vi "FDD Self TRAINING Polynomial APPLY FIT Ver02.vi"(7 "Polynomial ORDER\n(1st, 2nd, or 3rd)":i32=1, 9 "Which Model?\n(Row # = 0 to N)":i32=32, 10 "Independent Variables \n(3 values = Tid, Tidp, Tod)":dbl[](array[numeric])=[80.0, 60.5, 95.0], 11 "Coefficients with MSE File Path":path=path "C:/Vance/FDD Split System Project/FDD_LOW-HIGH_EfficiencyHP_Testing/Airtemp 16SEER/SHORT LINESET DATA/NF Cool Short/Airtemp-NF-Cool-Short-3rdOrder-FullCoeff.txt") -> (1 "ONLY Coefficients Array - Numeric":dbl[](array[numeric]) format="%_4p", 2 "Dependent Variable NAME":string, 3 "Calculated or Predicted VALUE":dbl)   [LabVIEW 2017]
uses:
  <vilib>/Utility/file.llb/Read Delimited Spreadsheet (string).vi
panel:
  in  "Tab Control":enum32{"INPUT Filename #1"}(tab)
  out "Coefficients Array - String":string[][](array[string])=[["ID_Xitron_Amps", "3.649182597E+0", "-5.140536303E-2", "2.881361728E-2", "-1.646757582E-2", "-2.402508606E-3", "6.602898885E-4", "4.179192017E-4", "1.267049882E-3", "6.501088333E-4", "-2.620550058E-4", "6.653976606E-6", "-1.708698056E-5", "8.692189159E-7", "-3.833312073E-6", "2.400456481E-5", "-8.196342284E-6", "-1.867608948E-6", "-8.415340803E-6", "5.486740068E-6", "1.699011560E-6", "9.690230426E-5", "6.880000000E+2", "1.963418024E+0", "1.932768441E-2"], ["ID_Xitron_Watts", "1.716229164E+2", "4.524054493E+0", "5.220102345E+0", "6.418177038E+0", "4.290692245E-2", "1.821805238E-2", "-1.124104457E-2", "-8.824969946E-2", "-1.166961761E-1", "-7.952292636E-2", "-1.422440795E-3", "-3.133902282E-3", "3.751462955E-4", "-5.178701767E-4", "2.536101609E-3", "-2.843734293E-5", "1.781301284E-3", "-1.484115870E-4", "1.368702178E-3", "3.084720061E-4", "6.243538110E+0", "6.880000000E+2", "1.963418024E+0", "4.906006925E+0"], ["OD_Xitron_Amps", "-2.013666809E+1", "5.895639722E-1", "-6.152918631E-1", "7.416404081E-1", "2.429300648E-2", "-3.985684156E-3", "1.199277373E-3", "-1.499044360E-2", "-5.428978683E-3", "-6.175574441E-3", "-8.599564404E-5", "1.423009400E-4", "-3.931088897E-7", "4.392436604E-5", "-2.108058706E-4", "5.559595816E-5", "-1.953419081E-5", "9.765111857E-5", "-3.027109034E-5", "1.631585602E-5", "8.721957263E-3", "6.880000000E+2", "1.963418024E+0", "1.833663966E-1"], ["OD_Xitron_Watts", "-6.618108354E+3", "1.891326198E+2", "-1.519041438E+2", "1.957588852E+2", "7.170307753E+0", "-9.645787016E-1", "1.489837836E-1", "-4.769126088E+0", "-1.974786395E+0", "-1.581263304E+0", "-2.906099271E-2", "3.417145482E-2", "-4.089114264E-4", "9.815585226E-3", "-5.541768764E-2", "1.721648401E-2", "2.694563150E-3", "2.858072095E-2", "-6.579645117E-3", "4.327883084E-3", "4.748946922E+2", "6.880000000E+2", "1.963418024E+0", "4.278696001E+1"], ["1500_ODLiqSV_TempF", "-4.585568082E+1", "-3.179944862E-1", "6.709568073E-1", "2.558442973E+0", "-4.709548642E-2", "-8.077274201E-2", "-8.182564700E-3", "6.900856647E-2", "2.520637506E-2", "1.959412419E-2", "5.772469079E-4", "-6.760434357E-4", "3.261229720E-4", "-1.822958171E-5", "4.383995310E-4", "-9.638001637E-5", "-2.762269210E-4", "-3.447483842E-4", "3.281085348E-4", "-1.568674968E-4", "3.605191728E-1", "6.880000000E+2", "1.963418024E+0", "1.178899969E+0"], ["1510_ODVapSV_TempF", "-2.524981499E+2", "3.035027022E+1", "-2.517284187E+0", "-1.349499227E+1", "3.021069222E-1", "2.235201575E-1", "-4.653221591E-2", "-6.587678304E-1", "-1.080220631E-1", "6.763840712E-2", "-7.302086758E-4", "3.834999590E-3", "-1.454390445E-3", "5.420993761E-4", "-4.426345241E-3", "5.802409144E-4", "5.233492767E-6", "3.808583702E-3", "-1.067181551E-3", "4.966372604E-5", "1.200077250E+0", "6.880000000E+2", "1.963418024E+0", "2.150885911E+0"], ["1526_Coriolis_IDSide_TempF", "-4.842315094E+1", "-1.103822645E-2", "3.773947647E-1", "2.588770976E+0", "-2.369077200E-2", "-8.280076735E-2", "-1.301817401E-2", "5.661397296E-2", "1.915600465E-2", "2.167109261E-2", "5.012325826E-4", "-5.938059862E-4", "3.075223820E-4", "3.011275874E-5", "2.667496862E-4", "-3.102377360E-5", "-2.587105277E-4", "-2.707606112E-4", "3.144593611E-4", "-1.699168272E-4", "3.367036994E-1", "6.880000000E+2", "1.963418024E+0", "1.139296380E+0"], ["1527_Coriolis_ODSide_TempF", "-5.243166565E+1", "1.029193229E-1", "9.742497441E-2", "2.826302948E+0", "-2.017037639E-3", "-8.593134019E-2", "-1.770234558E-2", "4.826595897E-2", "1.396850518E-2", "2.185245594E-2", "4.654432525E-4", "-5.437203584E-4", "3.009641069E-4", "7.553804404E-5", "1.063096855E-4", "1.096634779E-5", "-2.646547894E-4", "-2.080889222E-4", "3.223579627E-4", "-1.785506404E-4", "3.423572826E-1", "6.880000000E+2", "1.963418024E+0", "1.148821511E+0"], ["1600_IDVap_TempF", "-4.934301357E+2", "3.264320247E+1", "-2.450456574E+0", "-7.460325466E+0", "3.193026724E-1", "1.770472275E-1", "3.782493361E-2", "-6.704131915E-1", "-1.820543392E-1", "-7.019679136E-3", "-3.902996317E-4", "4.601575241E-3", "-1.267944176E-3", "3.035333565E-4", "-5.225256056E-3", "5.364605041E-4", "-5.465768990E-4", "4.062916107E-3", "-7.696228870E-4", "3.153040768E-4", "1.813312397E+0", "6.880000000E+2", "1.963418024E+0", "2.643924740E+0"], ["1601_IDLiq_TempF", "-4.844143438E+1", "-1.353672384E+0", "6.340211288E-1", "3.444826992E+0", "-6.479678449E-2", "-9.163893289E-2", "3.542190393E-3", "9.719177283E-2", "2.786507490E-2", "1.054005407E-2", "5.668761705E-4", "-7.055927749E-4", "4.053566153E-4", "-7.801185190E-5", "5.860490894E-4", "-1.169524253E-4", "-2.738485141E-4", "-5.022961589E-4", "3.245408642E-4", "-1.336724307E-4", "3.378593597E-1", "6.880000000E+2", "1.963418024E+0", "1.141249895E+0"], ["1602_ID2phase_Cool#1_TempF", "-2.066482712E+1", "2.196493252E+1", "-7.685685179E+0", "-1.189628617E+1", "6.594946945E-1", "1.214113511E-1", "-2.660448480E-1", "-6.263892498E-1", "-6.433460146E-2", "1.636241470E-1", "-7.528805413E-4", "2.690559273E-3", "-1.312521872E-3", "1.539626735E-3", "-6.085814059E-3", "1.103740516E-3", "3.629607856E-4", "3.949749020E-3", "-1.003220488E-3", "-5.598805433E-4", "4.129112078E-1", "6.880000000E+2", "1.963418024E+0", "1.261656441E+0"], ["1603_ID2Phase_Cool#2_TempF", "-4.015458109E+1", "2.280770805E+1", "-7.004230454E+0", "-1.227787951E+1", "6.260731973E-1", "1.176270768E-1", "-2.644515591E-1", "-6.234889761E-1", "-5.667946741E-2", "1.688356434E-1", "-5.731796195E-4", "2.560563959E-3", "-1.266847643E-3", "1.501411224E-3", "-5.874986140E-3", "1.003626875E-3", "2.919997628E-4", "3.928566670E-3", "-9.474044413E-4", "-5.825450754E-4", "3.877979605E-1", "6.880000000E+2", "1.963418024E+0", "1.222687673E+0"], ["1608_CompSuct_TempF", "-1.528094930E+2", "2.268345345E+1", "-1.023051056E+0", "-1.130267312E+1", "1.830036560E-1", "1.983583254E-1", "1.875691145E-3", "-4.950546158E-1", "-9.973535247E-2", "4.205611369E-2", "-6.233643553E-4", "3.071139618E-3", "-1.230773089E-3", "3.059749580E-4", "-3.099060472E-3", "4.172570843E-4", "-1.160275146E-4", "2.806841014E-3", "-7.131103906E-4", "1.289623237E-4", "9.760337296E-1", "6.880000000E+2", "1.963418024E+0", "1.939747436E+0"], ["1612_OD2PhaseHeat_F", "1.375343259E+2", "-1.904127868E+1", "6.911947135E+0", "7.356332861E+0", "-5.790635155E-1", "-1.147352753E-1", "1.644185127E-1", "5.583315256E-1", "1.246986298E-1", "-7.434084759E-2", "4.503154807E-4", "-6.333596685E-4", "1.003436680E-3", "-1.161049007E-3", "4.021066421E-3", "-6.130447944E-4", "1.039734667E-4", "-3.293007960E-3", "-4.350316849E-4", "2.344132111E-4", "1.983231695E-1", "6.880000000E+2", "1.963418024E+0", "8.743785612E-1"], ["1617_CompDisch_TempF", "-4.619956835E+2", "-2.796811999E+1", "7.558890200E+0", "3.599432317E+1", "-1.049328395E+0", "-2.112837974E-1", "6.513567757E-1", "9.196069356E-1", "6.552854782E-3", "-4.881903969E-1", "4.912137984E-4", "-1.121596795E-3", "2.282827065E-3", "-3.108662281E-3", "7.903435127E-3", "-1.686642956E-3", "-1.077725156E-3", "-5.559272560E-3", "9.706924146E-4", "1.804316884E-3", "3.519191250E+0", "6.880000000E+2", "1.963418024E+0", "3.683275532E+0"], ["1618_ID2Phase_Heat#2_F", "-1.828882612E+2", "2.509970551E+1", "-7.940743048E+0", "-8.422210484E+0", "8.744043084E-1", "1.655278777E-1", "-3.040610727E-1", "-7.805080692E-1", "-1.729566299E-1", "1.176670095E-1", "-2.019963728E-3", "3.708678881E-3", "-1.698173571E-3", "2.016372434E-3", "-7.534515923E-3", "1.770324385E-3", "7.482073657E-4", "4.749696506E-3", "-9.968740596E-4", "-3.827950439E-4", "9.121747188E-1", "6.880000000E+2", "1.963418024E+0", "1.875218113E+0"], ["1622_OD2PhaseCool_F", "-1.079342555E+2", "-5.681728059E+0", "-8.985853634E-1", "9.749367935E+0", "-1.187239790E-1", "-1.464367724E-2", "9.136074437E-2", "1.369001626E-1", "2.040683598E-2", "-1.168600191E-1", "9.787150928E-5", "4.920940653E-4", "6.320240761E-4", "-5.214726841E-4", "4.192037397E-4", "-6.977200405E-4", "-3.144420451E-5", "-4.815767216E-4", "-3.340869975E-4", "3.517868544E-4", "2.801887516E-1", "6.880000000E+2", "1.963418024E+0", "1.039293286E+0"], ["1630_ID2Phase_Heat#1_F", "1.036958015E+2", "1.854107232E+1", "-8.020385580E+0", "-1.292851450E+1", "5.907548840E-1", "1.423593049E-1", "-2.567838332E-1", "-5.666990955E-1", "-2.406262724E-2", "1.634546527E-1", "-1.028621256E-3", "2.194891794E-3", "-1.286210456E-3", "1.496264653E-3", "-5.163064752E-3", "1.045815743E-3", "5.088718207E-4", "3.491311260E-3", "-1.028752295E-3", "-5.551862467E-4", "4.653410073E-1", "6.880000000E+2", "1.963418024E+0", "1.339363428E+0"], ["1701_ODVapSV_psia", "-1.271507113E+2", "5.310358071E+1", "-1.955768746E+1", "-2.400134640E+1", "1.594268954E+0", "2.275501101E-1", "-5.951900834E-1", "-1.479095419E+0", "-1.843089529E-1", "3.564233424E-1", "-2.119399498E-3", "7.488742584E-3", "-2.760788831E-3", "3.551477869E-3", "-1.520052902E-2", "2.723027549E-3", "9.394153082E-4", "9.487891380E-3", "-2.727524957E-3", "-1.291668941E-3", "2.843216624E+0", "6.880000000E+2", "1.963418024E+0", "3.310684140E+0"], ["1702_ODLiqSV_psia", "-5.422342138E+2", "-1.159762766E+1", "-9.682897958E+0", "3.621663251E+1", "-2.044450193E-1", "-1.698402086E-1", "3.878130436E-1", "3.478059303E-1", "-5.770577163E-3", "-4.063691684E-1", "-7.496911760E-4", "9.895719005E-4", "1.421382637E-3", "-1.123470635E-3", "1.301987273E-3", "-4.470680195E-4", "-9.642171894E-4", "-1.771527599E-3", "-6.900656164E-5", "1.386338471E-3", "5.762628526E+0", "6.880000000E+2", "1.963418024E+0", "4.713278321E+0"], ["1707_IDVap_psia", "1.615316803E+1", "4.780594061E+1", "-1.545593179E+1", "-2.692720176E+1", "1.318538879E+0", "2.430331131E-1", "-5.470768080E-1", "-1.307845509E+0", "-1.197262601E-1", "3.648317280E-1", "-1.273587466E-3", "6.035640496E-3", "-2.661453376E-3", "3.112833691E-3", "-1.279419243E-2", "2.173173019E-3", "6.597065544E-4", "8.332254530E-3", "-2.269940886E-3", "-1.249089829E-3", "1.831320683E+0", "6.880000000E+2", "1.963418024E+0", "2.657020919E+0"], ["1710_ODSuctPort_psia", "5.025635613E+1", "5.002192336E+1", "-1.645924711E+1", "-2.924561169E+1", "1.405938578E+0", "2.767761540E-1", "-5.854707943E-1", "-1.392954167E+0", "-1.271941973E-1", "3.881228857E-1", "-1.348200830E-3", "6.082163940E-3", "-2.893492574E-3", "3.335508771E-3", "-1.337802658E-2", "2.262468565E-3", "6.860373423E-4", "8.828223314E-3", "-2.267542460E-3", "-1.314338024E-3", "2.069758435E+0", "6.880000000E+2", "1.963418024E+0", "2.824701783E+0"], ["1712_RotoMass_Massflow_lb/min", "-4.947722970E+1", "-3.775514116E+0", "-6.243587911E-1", "5.099321237E+0", "-6.647103644E-2", "-5.736972490E-2", "3.936854184E-2", "1.120381362E-1", "2.386415610E-2", "-4.352415740E-2", "2.096786191E-4", "1.114833845E-5", "3.710057398E-4", "-1.951028542E-4", "3.259716238E-4", "-1.557101471E-4", "-1.629776950E-4", "-5.233893635E-4", "-6.784336866E-5", "9.419508429E-5", "3.694656438E-2", "6.880000000E+2", "1.963418024E+0", "3.773981817E-1"], ["1713_RotoMass_Density_lbm/ft3", "6.972746898E+1", "5.329404135E-3", "-1.020933614E-3", "1.456172676E-3", "6.235853826E-5", "2.817350025E-5", "-7.354205153E-6", "-1.190081875E-4", "-1.498390594E-5", "-2.506210771E-5", "-3.415818956E-7", "8.689883626E-7", "-2.032567531E-7", "1.813567032E-7", "-8.362482712E-7", "1.932899152E-7", "6.608777585E-9", "6.614476248E-7", "-3.338571025E-7", "1.050118285E-7", "1.959109698E-7", "6.880000000E+2", "1.963418024E+0", "8.690447708E-4"], ["1724_IDLiq_psia", "-7.379310853E+2", "-2.817639301E+0", "-1.536492625E+1", "3.897973985E+1", "2.439076392E-1", "-1.509061218E-1", "2.953041679E-1", "4.267550291E-2", "-1.174240967E-1", "-4.142987132E-1", "-2.225403189E-3", "3.035192380E-3", "1.014478034E-3", "-3.088712310E-4", "-2.342670918E-3", "4.917734818E-4", "-4.737072015E-4", "1.402022438E-4", "-6.372076570E-4", "1.348374932E-3", "9.064058769E+0", "6.880000000E+2", "1.963418024E+0", "5.911179260E+0"], ["2219_NozTemp#1_F", "-1.754312882E+1", "1.374900200E+1", "-3.317343563E+0", "-7.770249170E+0", "3.179852436E-1", "1.037596492E-1", "-1.353724228E-1", "-3.643811409E-1", "-3.212616106E-2", "8.317630275E-2", "-5.199186267E-4", "1.729729139E-3", "-8.856288738E-4", "7.884642558E-4", "-3.186354143E-3", "6.139404982E-4", "2.404447950E-4", "2.194895571E-3", "-6.576816644E-4", "-2.204444687E-4", "1.566409833E-1", "6.880000000E+2", "1.963418024E+0", "7.770795388E-1"], ["2220_NozTemp#2_F", "-1.813162554E+1", "1.372464929E+1", "-3.329206860E+0", "-7.720651535E+0", "3.153119443E-1", "1.028214455E-1", "-1.340494561E-1", "-3.624910582E-1", "-3.119921692E-2", "8.260349684E-2", "-4.950354594E-4", "1.695214482E-3", "-8.807374944E-4", "7.835194513E-4", "-3.156630090E-3", "6.045147830E-4", "2.213202608E-4", "2.182689009E-3", "-6.389018610E-4", "-2.187143326E-4", "1.534357740E-1", "6.880000000E+2", "1.963418024E+0", "7.690880929E-1"], ["Exit TC Grid AVG Temp (F)", "2.499177681E+1", "1.313499641E+1", "-1.579284719E+0", "-9.751778296E+0", "2.359287146E-1", "1.185207521E-1", "-1.133913691E-1", "-3.336428953E-1", "-2.706899567E-2", "9.142140009E-2", "-6.137909095E-4", "1.874317129E-3", "-8.759602864E-4", "6.200158032E-4", "-2.701478540E-3", "5.373648669E-4", "3.741687163E-4", "1.966048660E-3", "-8.066352292E-4", "-2.146806852E-4", "1.296028769E-1", "6.880000000E+2", "1.963418024E+0", "7.068383339E-1"], ["TC Grid  DT Temp (F)", "-4.257854183E+1", "-9.590738646E+0", "1.478875346E+0", "8.352663558E+0", "-3.728266342E-1", "-1.110798530E-1", "2.543815249E-1", "3.488619787E-1", "1.191094500E-3", "-1.219780037E-1", "9.010565418E-5", "-1.961396831E-3", "1.173883695E-3", "-1.402270925E-3", "3.985703674E-3", "-7.725970486E-4", "-1.974511799E-6", "-2.262454546E-3", "8.308079870E-4", "4.062025873E-4", "4.479560438E-1", "6.880000000E+2", "1.963418024E+0", "1.314106228E+0"], ["AVG Nozzle Temp (F)", "-1.783734967E+1", "1.373682483E+1", "-3.323275076E+0", "-7.745450706E+0", "3.166485628E-1", "1.032905394E-1", "-1.347109186E-1", "-3.634360716E-1", "-3.166268813E-2", "8.288990059E-2", "-5.074770197E-4", "1.712471779E-3", "-8.831831306E-4", "7.859917415E-4", "-3.171491893E-3", "6.092276189E-4", "2.308825109E-4", "2.188792115E-3", "-6.482917459E-4", "-2.195793956E-4", "1.549526808E-1", "6.880000000E+2", "1.963418024E+0", "7.728804477E-1"], ["AVG Noz DP (in H2O)", "-1.137797681E+0", "1.139881567E-1", "-4.855784009E-2", "1.778732377E-2", "2.341579537E-3", "-5.339749034E-5", "-1.255346805E-4", "-2.466438349E-3", "-5.517348287E-4", "-1.204757019E-4", "-8.404469252E-6", "-1.104968660E-6", "-4.258171433E-7", "1.715886404E-6", "-1.068197014E-5", "3.957447596E-6", "4.043993108E-6", "1.263395541E-5", "1.739848601E-6", "1.336642894E-7", "4.743755967E-5", "6.880000000E+2", "1.963418024E+0", "1.352302787E-2"], ["Unit ESP (in H2O)", "-3.439738970E+0", "2.916621869E-1", "-1.240495672E-1", "-3.041133172E-2", "5.885990550E-3", "-4.074613399E-4", "-5.756427155E-4", "-6.075054737E-3", "-1.119043745E-3", "7.007862690E-4", "-1.667015324E-5", "1.651625482E-8", "-1.637373039E-6", "3.626950987E-6", "-3.123506980E-5", "1.104404076E-5", "1.016745289E-5", "3.178763763E-5", "1.637571913E-6", "-2.961992416E-6", "2.398511109E-4", "6.880000000E+2", "1.963418024E+0", "3.040770481E-2"], ["Indoor Unit SCFM", "-7.335853432E+0", "3.749046443E+1", "-2.818193672E+0", "1.931921094E+1", "-2.294186759E-1", "-1.787247292E-1", "2.855866698E-1", "-3.375291253E-1", "-4.240954599E-2", "-2.309628818E-1", "-6.426877515E-4", "-7.668786554E-3", "1.823057108E-3", "-1.104643875E-3", "7.229583417E-3", "-9.636155661E-4", "-5.625477236E-5", "3.089714452E-4", "3.740617520E-3", "5.791876535E-4", "1.744373054E+1", "6.880000000E+2", "1.963418024E+0", "8.200351306E+0"], ["Indoor Unit CFM", "5.870901161E+1", "8.838692813E+1", "-5.113773977E+1", "9.405102985E-1", "2.801213135E+0", "1.122477420E-1", "-3.965379432E-1", "-2.376335379E+0", "-5.733522956E-1", "8.559257420E-2", "-8.812479176E-3", "6.164455892E-3", "-2.165085942E-3", "2.852821761E-3", "-1.864415606E-2", "5.286769922E-3", "4.632039322E-3", "1.352960052E-2", "-1.706240441E-3", "-3.905071358E-4", "3.145326437E+1", "6.880000000E+2", "1.963418024E+0", "1.101147852E+1"], ["Sensible Capacity (Btu/h)", "-9.575239359E+4", "-1.294536948E+4", "1.905086089E+3", "1.265908979E+4", "-5.378583272E+2", "-1.635344460E+2", "3.697621314E+2", "4.932746269E+2", "3.061895457E+0", "-1.822635301E+2", "2.058180973E-1", "-2.958783615E+0", "1.720283557E+0", "-2.023987174E+0", "5.796953442E+0", "-1.158494644E+0", "-6.877770687E-2", "-3.213286283E+0", "1.286961793E+0", "6.019894048E-1", "8.591656358E+5", "6.880000000E+2", "1.963418024E+0", "1.819915494E+3"], ["Latent Capacity (Btu/h)", "-1.613809630E+5", "-9.924934542E+1", "-7.112672363E+2", "5.672008031E+3", "-2.210236246E+2", "-2.203800999E+1", "5.895196575E+1", "9.658382518E+1", "1.223361300E+2", "-6.982281156E+1", "1.924945356E+0", "5.985960021E-1", "1.967482386E-1", "-2.646350109E-1", "-1.249715862E-1", "-8.319681059E-1", "-1.359122700E+0", "-9.301681808E-2", "-2.254308371E-1", "2.472010209E-1", "8.962121847E+5", "6.880000000E+2", "1.963418024E+0", "1.858738076E+3"], ["TOTAL Capacity (Btu/h)", "-2.571333565E+5", "-1.304461883E+4", "1.193818849E+3", "1.833109782E+4", "-7.588819518E+2", "-1.855724560E+2", "4.287140971E+2", "5.898584521E+2", "1.253980255E+2", "-2.520863417E+2", "2.130763453E+0", "-2.360187615E+0", "1.917031796E+0", "-2.288622185E+0", "5.671981856E+0", "-1.990462750E+0", "-1.427900407E+0", "-3.306303101E+0", "1.061530957E+0", "8.491904258E-1", "9.226341900E+5", "6.880000000E+2", "1.963418024E+0", "1.885938583E+3"], ["SHR", "1.409496581E+0", "-5.315813104E-1", "5.305446081E-2", "3.732189749E-1", "-9.538459857E-3", "-5.387729077E-3", "7.413719359E-3", "1.444159300E-2", "-1.323440633E-3", "-4.104652237E-3", "-2.791338927E-5", "-7.706918986E-5", "4.468436884E-5", "-4.215603811E-5", "1.396978807E-4", "-8.270449144E-6", "2.022935805E-5", "-9.699612686E-5", "3.204577950E-5", "1.139932919E-5", "7.667089070E-4", "6.880000000E+2", "1.963418024E+0", "5.436608099E-2"], ["ODVapSV_Suph_F", "-1.531685671E+2", "7.736125102E+0", "5.496257324E+0", "-3.831114058E+0", "-3.658565402E-1", "1.253264058E-1", "2.042712961E-1", "-3.416551092E-2", "-3.120034254E-2", "-7.719138247E-2", "1.433280389E-4", "8.685130214E-4", "-2.772884354E-4", "-9.705029207E-4", "1.836149520E-3", "-5.563934051E-4", "-3.484705855E-4", "-1.600846766E-4", "-1.082111631E-5", "5.747559901E-4", "1.466487551E+0", "6.880000000E+2", "1.963418024E+0", "2.377672111E+0"], ["ODVapSV_Tsat_F", "-9.932961364E+1", "2.261414618E+1", "-8.013541192E+0", "-9.663878230E+0", "6.679634583E-1", "9.819376864E-2", "-2.508035217E-1", "-6.246023430E-1", "-7.682171584E-2", "1.448297857E-1", "-8.735367507E-4", "2.966486689E-3", "-1.177102087E-3", "1.512602327E-3", "-6.262494796E-3", "1.136634316E-3", "3.537041316E-4", "3.968668494E-3", "-1.056360543E-3", "-5.250922350E-4", "4.597261742E-1", "6.880000000E+2", "1.963418024E+0", "1.331258485E+0"], ["ODLiqSV_Tsat_F", "-1.695480861E+2", "-3.791180368E+0", "-1.577375499E+0", "1.079483774E+1", "-8.295583575E-2", "-5.296622944E-2", "1.005231365E-1", "1.171244146E-1", "7.032719084E-4", "-1.132741136E-1", "-8.780386147E-5", "1.453020048E-4", "4.455193121E-4", "-3.667343510E-4", "5.597909886E-4", "-1.845359755E-4", "-2.104028951E-4", "-6.082820082E-4", "6.144653732E-6", "3.573211894E-4", "2.656341209E-1", "6.880000000E+2", "1.963418024E+0", "1.011939861E+0"], ["ODLiqSV_Tsub_F", "-1.236923822E+2", "-3.473185910E+0", "-2.248331979E+0", "8.236393766E+0", "-3.586032918E-2", "2.780652564E-2", "1.087056897E-1", "4.811583354E-2", "-2.450311258E-2", "-1.328682286E-1", "-6.650509763E-4", "8.213457362E-4", "1.193962742E-4", "-3.485047271E-4", "1.213912052E-4", "-8.815588413E-5", "6.582418640E-5", "-2.635335246E-4", "-3.219640274E-4", "5.141886621E-4", "1.009382009E+0", "6.880000000E+2", "1.963418024E+0", "1.972606924E+0"], ["1612_OD2phase_Heating_F", "1.375343259E+2", "-1.904127868E+1", "6.911947135E+0", "7.356332861E+0", "-5.790635155E-1", "-1.147352753E-1", "1.644185127E-1", "5.583315256E-1", "1.246986298E-1", "-7.434084759E-2", "4.503154807E-4", "-6.333596685E-4", "1.003436680E-3", "-1.161049007E-3", "4.021066421E-3", "-6.130447944E-4", "1.039734667E-4", "-3.293007960E-3", "-4.350316849E-4", "2.344132111E-4", "1.983231695E-1", "6.880000000E+2", "1.963418024E+0", "8.743785612E-1"], ["1622_OD2phase_Cooling_F", "-1.079342555E+2", "-5.681728059E+0", "-8.985853634E-1", "9.749367935E+0", "-1.187239790E-1", "-1.464367724E-2", "9.136074437E-2", "1.369001626E-1", "2.040683598E-2", "-1.168600191E-1", "9.787150928E-5", "4.920940653E-4", "6.320240761E-4", "-5.214726841E-4", "4.192037397E-4", "-6.977200405E-4", "-3.144420451E-5", "-4.815767216E-4", "-3.340869975E-4", "3.517868544E-4", "2.801887516E-1", "6.880000000E+2", "1.963418024E+0", "1.039293286E+0"], ["1710_CompSuct_psia", "5.025635613E+1", "5.002192336E+1", "-1.645924711E+1", "-2.924561169E+1", "1.405938578E+0", "2.767761540E-1", "-5.854707943E-1", "-1.392954167E+0", "-1.271941973E-1", "3.881228857E-1", "-1.348200830E-3", "6.082163940E-3", "-2.893492574E-3", "3.335508771E-3", "-1.337802658E-2", "2.262468565E-3", "6.860373423E-4", "8.828223314E-3", "-2.267542460E-3", "-1.314338024E-3", "2.069758435E+0", "6.880000000E+2", "1.963418024E+0", "2.824701783E+0"], ["CompSuct_TempF", "-1.528094930E+2", "2.268345345E+1", "-1.023051056E+0", "-1.130267312E+1", "1.830036560E-1", "1.983583254E-1", "1.875691145E-3", "-4.950546158E-1", "-9.973535247E-2", "4.205611369E-2", "-6.233643553E-4", "3.071139618E-3", "-1.230773089E-3", "3.059749580E-4", "-3.099060472E-3", "4.172570843E-4", "-1.160275146E-4", "2.806841014E-3", "-7.131103906E-4", "1.289623237E-4", "9.760337296E-1", "6.880000000E+2", "1.963418024E+0", "1.939747436E+0"], ["CompSuct_Suph_F", "-1.340849531E+2", "1.552772665E+0", "5.795097431E+0", "5.883809093E-1", "-4.037199694E-1", "8.091812283E-2", "2.472291050E-1", "8.887894393E-2", "-4.934879950E-2", "-1.166015906E-1", "-5.477045901E-5", "6.352853249E-4", "-1.064105490E-5", "-1.102997392E-3", "2.418734469E-3", "-5.272020758E-4", "-3.825618854E-4", "-8.687979975E-4", "1.998307055E-4", "6.662056741E-4", "1.229631082E+0", "6.880000000E+2", "1.963418024E+0", "2.177209345E+0"], ["CompSuct_Tsat_F", "-1.872454573E+1", "2.113068173E+1", "-6.818149392E+0", "-1.189105404E+1", "5.867236285E-1", "1.174402184E-1", "-2.453534060E-1", "-5.839335832E-1", "-5.038654486E-2", "1.586576953E-1", "-5.685937675E-4", "2.435853951E-3", "-1.220132075E-3", "1.408972300E-3", "-5.517794786E-3", "9.444590541E-4", "2.665342960E-4", "3.675639121E-3", "-9.129409524E-4", "-5.372432956E-4", "3.467028339E-1", "6.880000000E+2", "1.963418024E+0", "1.156089533E+0"], ["CompDisch_psia", "-5.422342138E+2", "-1.159762766E+1", "-9.682897958E+0", "3.621663251E+1", "-2.044450193E-1", "-1.698402086E-1", "3.878130436E-1", "3.478059303E-1", "-5.770577163E-3", "-4.063691684E-1", "-7.496911760E-4", "9.895719005E-4", "1.421382637E-3", "-1.123470635E-3", "1.301987273E-3", "-4.470680195E-4", "-9.642171894E-4", "-1.771527599E-3", "-6.900656164E-5", "1.386338471E-3", "5.762628526E+0", "6.880000000E+2", "1.963418024E+0", "4.713278321E+0"], ["1617_CompDisch_TempF", "-4.619956835E+2", "-2.796811999E+1", "7.558890200E+0", "3.599432317E+1", "-1.049328395E+0", "-2.112837974E-1", "6.513567757E-1", "9.196069356E-1", "6.552854782E-3", "-4.881903969E-1", "4.912137984E-4", "-1.121596795E-3", "2.282827065E-3", "-3.108662281E-3", "7.903435127E-3", "-1.686642956E-3", "-1.077725156E-3", "-5.559272560E-3", "9.706924146E-4", "1.804316884E-3", "3.519191250E+0", "6.880000000E+2", "1.963418024E+0", "3.683275532E+0"], ["CompDisch_Suph_F", "-2.925827467E+2", "-2.417600442E+1", "9.133805026E+0", "2.519885952E+1", "-9.662875471E-1", "-1.582919624E-1", "5.508231642E-1", "8.024239119E-1", "5.848799247E-3", "-3.749389603E-1", "5.786602502E-4", "-1.266756848E-3", "1.837049851E-3", "-2.741621942E-3", "7.343150387E-3", "-1.501847674E-3", "-8.674450003E-4", "-4.950702581E-3", "9.645379653E-4", "1.447192086E-3", "2.463784998E+0", "6.880000000E+2", "1.963418024E+0", "3.081869016E+0"], ["CompDisch_Tsat_F", "-1.694129093E+2", "-3.792115026E+0", "-1.574914602E+0", "1.079546212E+1", "-8.304084171E-2", "-5.299181839E-2", "1.005336086E-1", "1.171830038E-1", "7.040499837E-4", "-1.132514255E-1", "-8.744658514E-5", "1.451600711E-4", "4.457771428E-4", "-3.670403291E-4", "5.602847449E-4", "-1.847952550E-4", "-2.102800637E-4", "-6.085698979E-4", "6.154437114E-6", "3.571247740E-4", "2.654244699E-1", "6.880000000E+2", "1.963418024E+0", "1.011540446E+0"], ["Refrig-Side Capacity_Btu/h", "-2.545361196E+5", "-1.933874326E+4", "-1.691551366E+3", "2.526788105E+4", "-3.929117778E+2", "-2.507092264E+2", "2.360320145E+2", "5.711951068E+2", "1.008249715E+2", "-2.430265178E+2", "8.147131932E-1", "2.069505690E-1", "1.791752730E+0", "-1.193649099E+0", "2.071187972E+0", "-8.658581461E-1", "-6.764703276E-1", "-2.760995386E+0", "-3.598132097E-1", "6.256628833E-1", "7.734237509E+5", "6.880000000E+2", "1.963418024E+0", "1.726718435E+3"], ["IDLiq@TXV_Tsat_F", "-2.195384759E+2", "-1.444944555E+0", "-2.807925177E+0", "1.129148253E+1", "2.490310461E-2", "-4.382800050E-2", "7.493409718E-2", "3.755061073E-2", "-2.616821150E-2", "-1.141182362E-1", "-4.071177131E-4", "6.492798586E-4", "3.238373038E-4", "-1.696134622E-4", "-3.433590188E-4", "2.749820935E-5", "-8.915693852E-5", "-1.089492776E-4", "-1.376855970E-4", "3.503565652E-4", "4.039700959E-1", "6.880000000E+2", "1.963418024E+0", "1.247921831E+0"], ["IDLiq@TXV_Tsub_F", "-1.710970854E+2", "-9.126850595E-2", "-3.441946765E+0", "7.846654376E+0", "8.969996120E-2", "4.781094846E-2", "7.139188230E-2", "-5.964125108E-2", "-5.403330499E-2", "-1.246582762E-1", "-9.739941629E-4", "1.354872800E-3", "-8.151946507E-5", "-9.160147507E-5", "-9.294085678E-4", "1.444508213E-4", "1.846917602E-4", "3.933473347E-4", "-4.622265177E-4", "4.840289567E-4", "1.230292577E+0", "6.880000000E+2", "1.963418024E+0", "2.177794894E+0"], ["IDVap_Suph_F", "-4.609486691E+2", "1.255642026E+1", "3.859272995E+0", "3.423801646E+0", "-2.243953864E-1", "7.409475948E-2", "2.646670209E-1", "-1.264606199E-1", "-1.354543238E-1", "-1.548129318E-1", "1.429221052E-4", "2.219176471E-3", "-1.527350979E-4", "-9.999740044E-4", "-1.830561674E-5", "-3.622936998E-4", "-7.982249998E-4", "6.288128842E-4", "1.322823748E-4", "8.205674934E-4", "2.120976931E+0", "6.880000000E+2", "1.963418024E+0", "2.859438405E+0"], ["IDVap_Tsat_F", "-3.248146899E+1", "2.008678244E+1", "-6.309729546E+0", "-1.088412723E+1", "5.436980787E-1", "1.029524844E-1", "-2.268420965E-1", "-5.439525928E-1", "-4.660002157E-2", "1.477932505E-1", "-5.332219795E-4", "2.382398929E-3", "-1.115209126E-3", "1.303507403E-3", "-5.206950557E-3", "8.987542433E-4", "2.516482706E-4", "3.434103337E-3", "-9.019053792E-4", "-5.052634053E-4", "3.005119595E-1", "6.880000000E+2", "1.963418024E+0", "1.076325560E+0"], ["CoriolisLiq_ID#1_Tsub_F", "-1.711153724E+2", "-1.433903936E+0", "-3.185320571E+0", "8.702711659E+0", "4.859392971E-2", "3.897277726E-2", "8.795223899E-2", "-1.906342389E-2", "-4.532421278E-2", "-1.357893238E-1", "-9.083501853E-4", "1.243085910E-3", "1.631478801E-5", "-1.997260487E-4", "-6.101091650E-4", "5.852203811E-5", "1.695535219E-4", "1.618117116E-4", "-4.521449833E-4", "5.202733727E-4", "1.232563118E+0", "6.880000000E+2", "1.963418024E+0", "2.179803560E+0"], ["CoriolisLiq_OD#2_Tsub_F", "-1.171164164E+2", "-3.894099723E+0", "-1.674800085E+0", "7.968534457E+0", "-8.093881395E-2", "3.296511348E-2", "1.182254796E-1", "6.885846056E-2", "-1.326522782E-2", "-1.351265665E-1", "-5.532469856E-4", "6.890223262E-4", "1.445551716E-4", "-4.422723967E-4", "4.534813670E-4", "-1.955023475E-4", "5.425183569E-5", "-4.001931168E-4", "-3.162132978E-4", "5.358718284E-4", "9.463956945E-1", "6.880000000E+2", "1.963418024E+0", "1.910069419E+0"], ["Blower_Heat_Btu/h", "5.855773907E+2", "1.543607393E+1", "1.781098920E+1", "2.189882005E+1", "1.463984194E-1", "6.215999473E-2", "-3.835444409E-2", "-3.011079746E-1", "-3.981673529E-1", "-2.713322247E-1", "-4.853367992E-3", "-1.069287459E-2", "1.279999160E-3", "-1.766973043E-3", "8.653178690E-3", "-9.702821406E-5", "6.077799981E-3", "-5.063803347E-4", "4.670011832E-3", "1.052506485E-3", "7.268567233E+1", "6.880000000E+2", "1.963418024E+0", "1.673929563E+1"], ["Adj_RefSide_Q_Btu/h", "-2.551216971E+5", "-1.935417935E+4", "-1.709362350E+3", "2.524598224E+4", "-3.930581761E+2", "-2.507713865E+2", "2.360703688E+2", "5.714962149E+2", "1.012231389E+2", "-2.427551855E+2", "8.195665604E-1", "2.176434451E-1", "1.790472732E+0", "-1.191882126E+0", "2.062534792E+0", "-8.657611172E-1", "-6.825481264E-1", "-2.760489007E+0", "-3.644832228E-1", "6.246103765E-1", "7.799978000E+5", "6.880000000E+2", "1.963418024E+0", "1.734041401E+3"], ["COP", "-2.237422820E+1", "-2.006160170E+0", "3.845570213E-1", "2.177207477E+0", "-9.755528939E-2", "-2.330712453E-2", "4.889353046E-2", "7.989071092E-2", "1.712595992E-2", "-2.933830713E-2", "2.698786334E-4", "-3.328218649E-4", "2.316797558E-4", "-2.695505600E-4", "7.495906407E-4", "-2.393156071E-4", "-1.701958633E-4", "-4.539659092E-4", "1.388851460E-4", "9.853982773E-5", "9.810289504E-3", "6.880000000E+2", "1.963418024E+0", "1.944704796E-1"], ["SCFM/TON", "2.455025009E+4", "3.115259398E+3", "-5.014085972E+2", "-2.940604234E+3", "8.074506047E+1", "3.111805892E+1", "-3.960570057E+1", "-9.290190901E+1", "-1.108955267E+1", "3.122193608E+1", "-1.250870592E-1", "2.355015576E-1", "-2.515316290E-1", "2.173017506E-1", "-6.506671942E-1", "1.524076341E-1", "7.720638828E-2", "5.233469183E-1", "-8.089481961E-2", "-8.860805990E-2", "1.023790810E+4", "6.880000000E+2", "1.963418024E+0", "1.986636392E+2"], ["ODAir_Exit_TempF", "-5.045051727E+1", "-1.021755477E+1", "1.853451132E+0", "9.784387973E+0", "-3.037557867E-1", "-1.063198454E-1", "1.378800428E-1", "3.236224866E-1", "5.352116366E-2", "-9.373435201E-2", "4.688536253E-4", "-6.657783717E-4", "8.350349652E-4", "-8.283972436E-4", "2.255287598E-3", "-5.038059967E-4", "-1.891893231E-4", "-1.827006539E-3", "1.055377137E-4", "2.812255200E-4", "1.247708707E-1", "6.880000000E+2", "1.963418024E+0", "6.935365860E-1"], ["ODAir_DT(F)", "-5.045051727E+1", "-1.021755477E+1", "1.853451132E+0", "8.784387973E+0", "-3.037557867E-1", "-1.063198454E-1", "1.378800428E-1", "3.236224866E-1", "5.352116366E-2", "-9.373435201E-2", "4.688536253E-4", "-6.657783717E-4", "8.350349652E-4", "-8.283972436E-4", "2.255287598E-3", "-5.038059967E-4", "-1.891893231E-4", "-1.827006539E-3", "1.055377137E-4", "2.812255200E-4", "1.247708707E-1", "6.880000000E+2", "1.963418024E+0", "6.935365860E-1"], ["LiqLine_DP(psid)", "1.956968715E+2", "-8.779988360E+0", "5.682028296E+0", "-2.763107338E+0", "-4.483526585E-1", "-1.893408673E-2", "9.250887569E-2", "3.051304274E-1", "1.116535196E-1", "7.929544805E-3", "1.475712013E-3", "-2.045620479E-3", "4.069046031E-4", "-8.145994043E-4", "3.644658191E-3", "-9.388415014E-4", "-4.905099879E-4", "-1.911729843E-3", "5.682010954E-4", "3.796353865E-5", "6.845796271E-1", "6.880000000E+2", "1.963418024E+0", "1.624518864E+0"]]
  out "Dependent Variable NAME 2":string
  out "Coefficient HEADER LABELS - String":string[](array[string])
  # "Multivariate Polynomial APPLY FIT for 3 Independent Variables"
  # "y = a0*y0 + a1*y1 + .....+ai*yi  \nwhere i =0 to 19.\ny0=1;\ny1=x1;\ny2=x2;              1st Order\ny3=x3;\n--------------\ny4=x1*x2;\ny5=x1*x3;\ny6=x2*x3;\ny7=x1**2;        2nd Order\ny8=x2**2;\ny9=x3**2;\n----------------\ny10=x1*x2*x3;\ny11=x1*x2**2;\ny12=x1*x3**2;\ny13=x2*x3**2;\ny14=x1**2*x2;  3rd Order\ny15=x1**2*x3;\ny16=x2**2*x3;\ny17=x1**3;\ny18=x2**3;\ny19=x3**3;"
  # "x1"
  # "x2"
  # "x3"
  # "a0 ---->---------------------------------------------------------->---------------------------------------------->--------------------------------------------------->---------------------------------------->--a19"
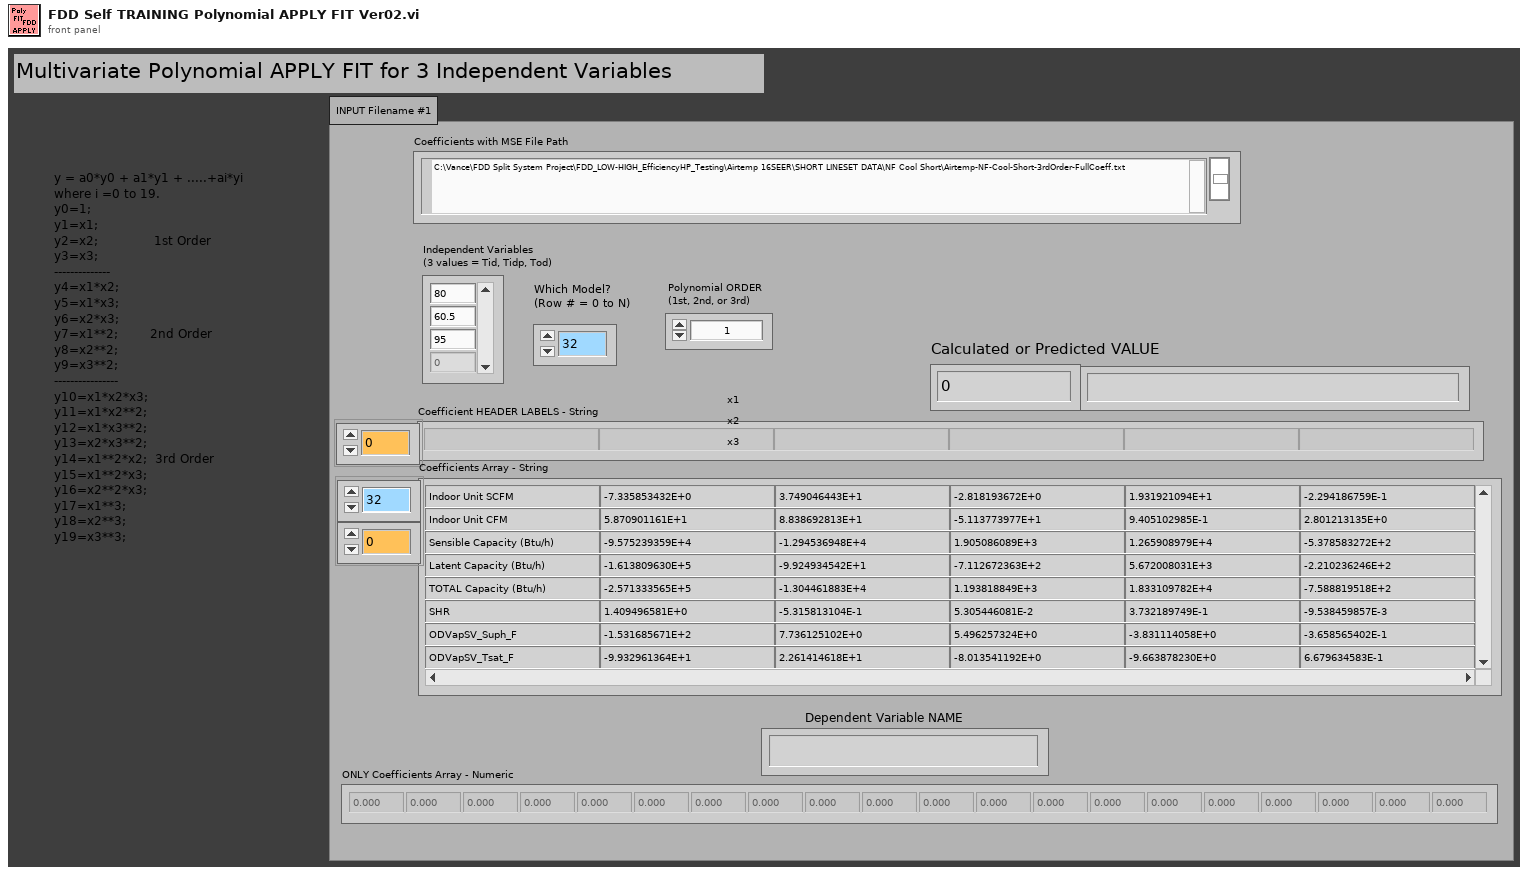
[diagram p1: front panel]
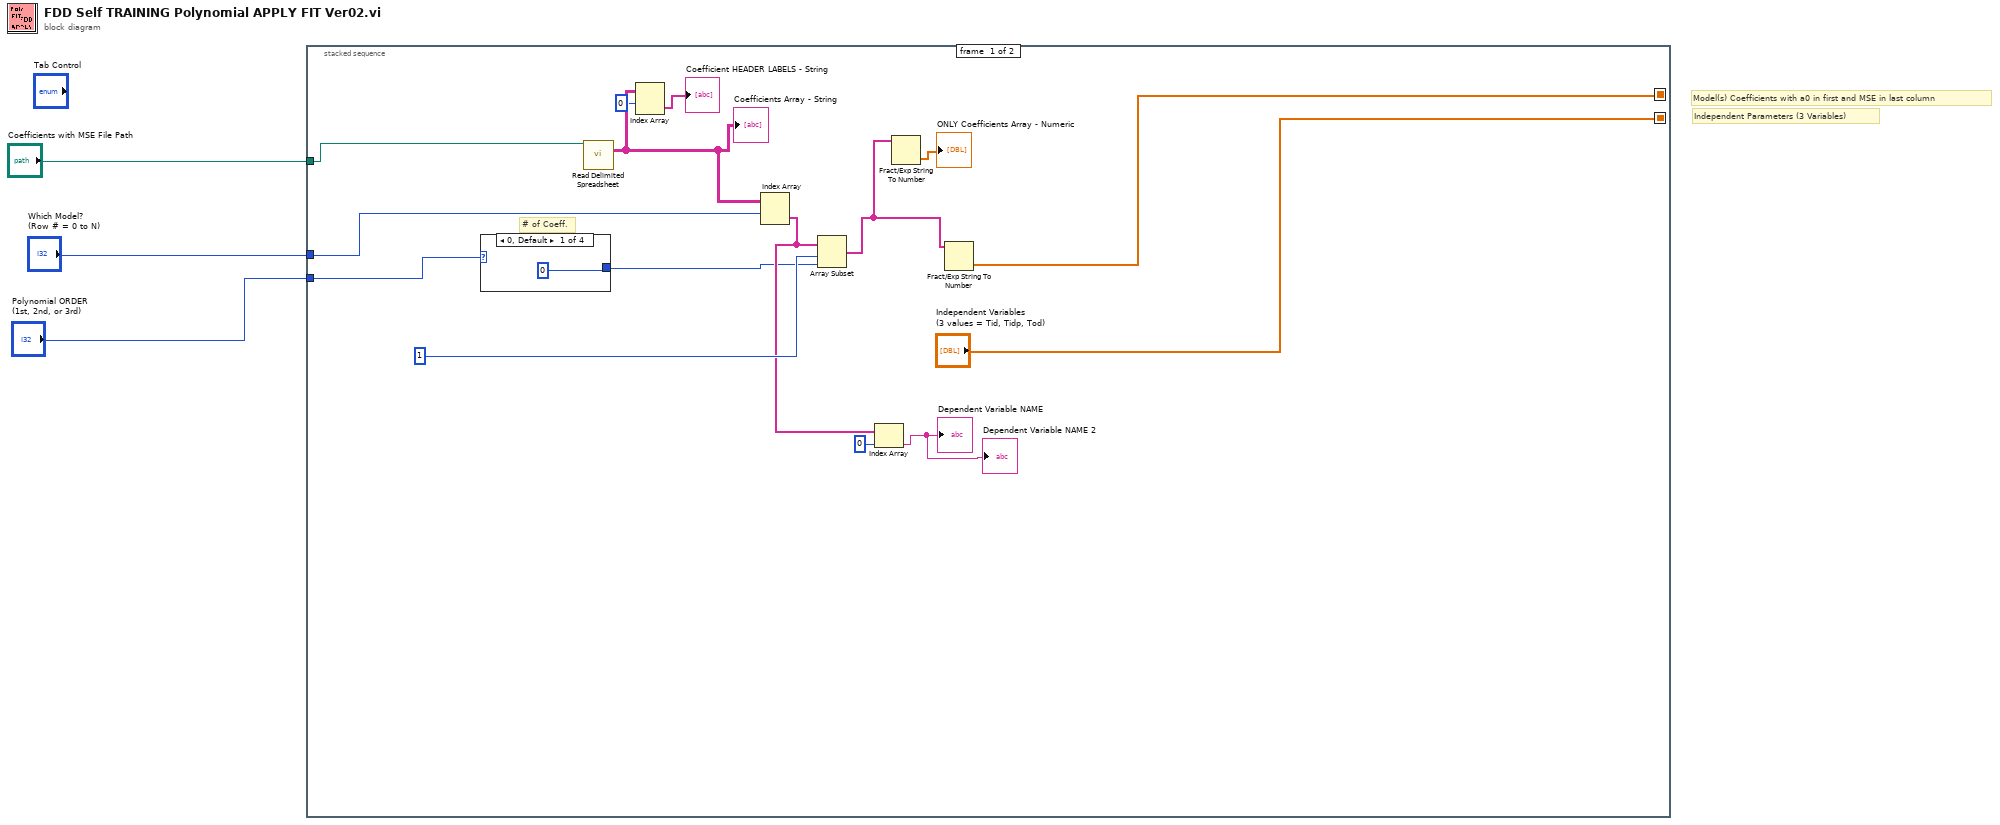
[diagram p0: block diagram]
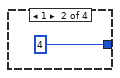
[diagram p2: hidden frame]
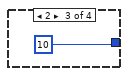
[diagram p3: hidden frame]
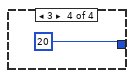
[diagram p4: hidden frame]
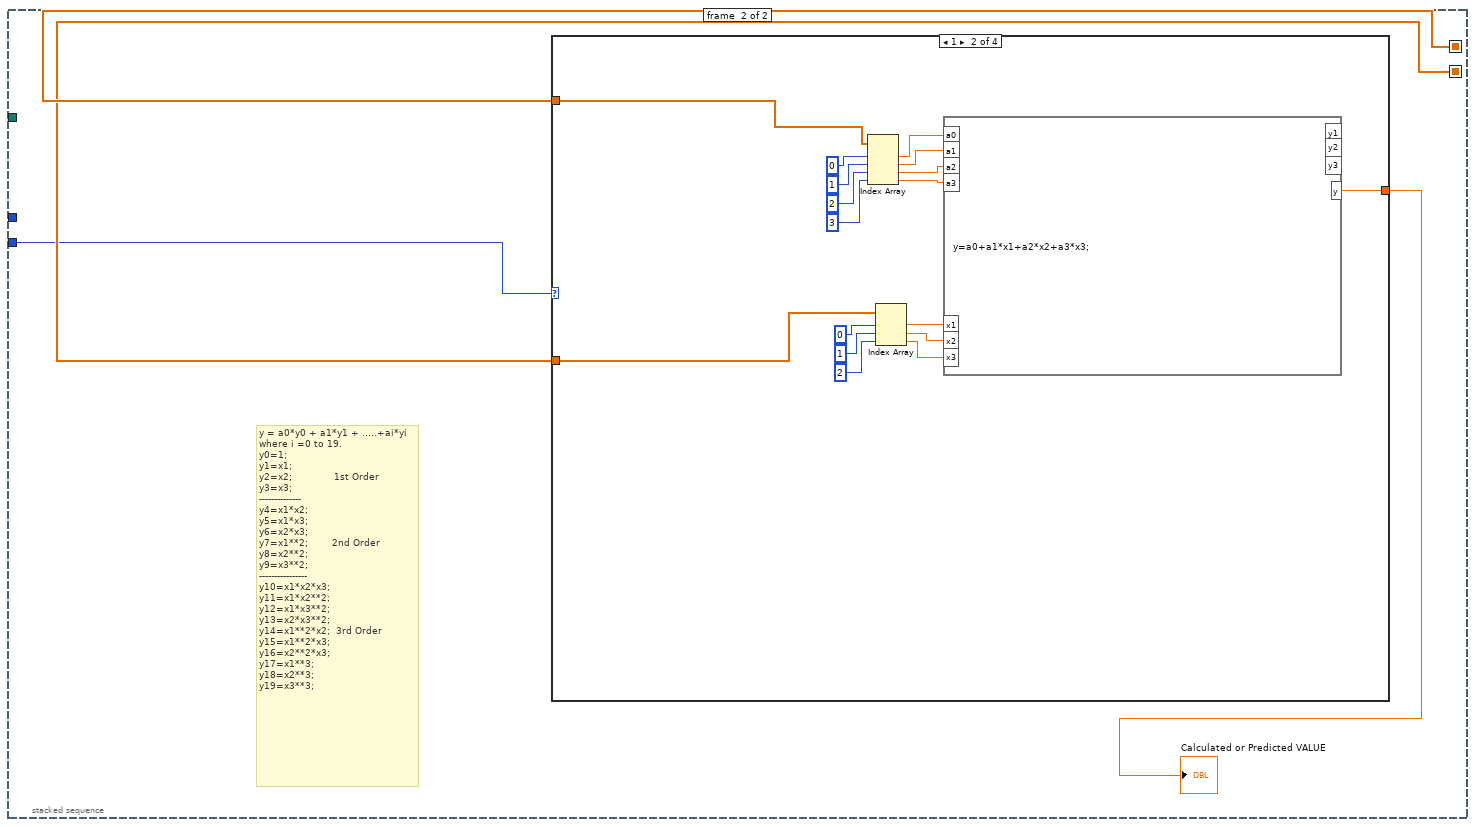
[diagram p5: hidden frame]
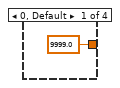
[diagram p6: hidden frame]
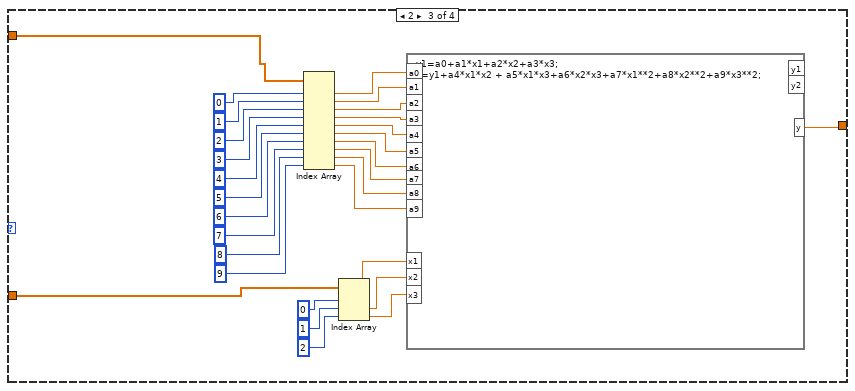
[diagram p7: hidden frame]
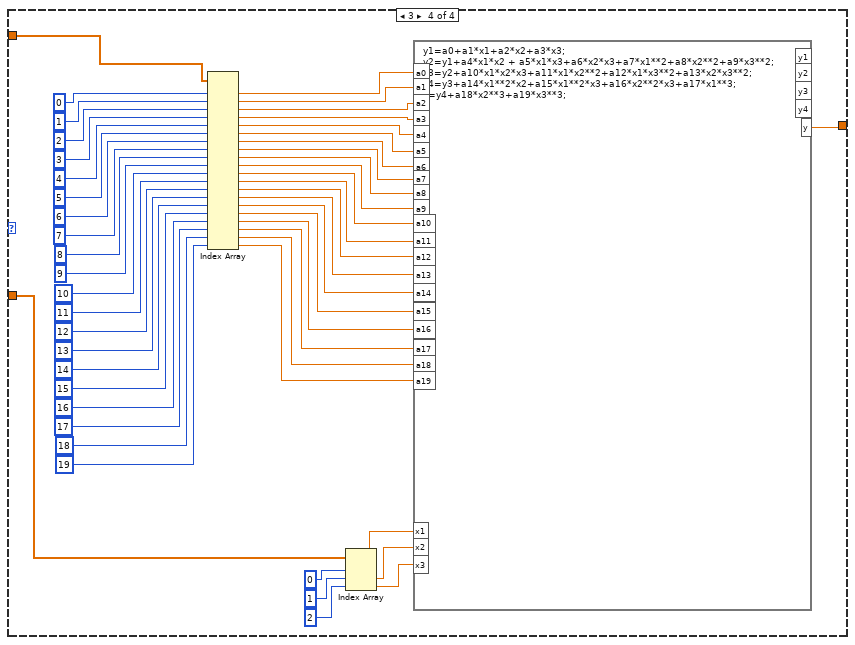
[diagram p8: hidden frame]
diagram:
  # "Independent Parameters (3 Variables)"
  # "Model(s) Coefficients with a0 in first and MSE in last column"
  n1 = stacked-sequence {
    seq-local: [w17 _] -> [_ w25]
    seq-local: ["Independent Variables \n(3 values = Tid, Tidp, Tod)" _] -> [_ w24]
    tunnel: "Which Model?\n(Row # = 0 to N)" -> [w15 _]
    tunnel: "Coefficients with MSE File Path" -> [w18 _]
    tunnel: "Polynomial ORDER\n(1st, 2nd, or 3rd)" -> [w5 w23]
    frame #0 {
      # "# of Coeff."
      n2 = case shown="0, Default" w5 {
        tunnel: [0 ("a0 - First Coef. COLUMN index") 4 ("a0 - First Coef. COLUMN index") 10 ("a0 - First Coef. COLUMN index") 20 ("a0 - First Coef. COLUMN index")] -> w4
        frame 0, Default {
        }
        frame 1 {
        }
        frame 2 {
        }
        frame 3 {
        }
      }
      n3 = call-poly <vilib>:"Read Delimited Spreadsheet.vi"("file path (dialog if empty)"=w18) -> ("all rows"=w8:string[][])  [unwired: 9 in, 5 out]
      "Coefficients Array - String" <- w8
      n4 = Index Array(array=w8, index (row)=0) -> (element=→"Coefficient HEADER LABELS - String":string[])  [unwired: 1 in]
      n5 = Index Array(array=w8, index (row)=w15) -> (element=w13:string[])  [unwired: 1 in]
      n6 = Array Subset(array=w13, index=1 ("a0 - First Coef. COLUMN index"), length=w4) -> (w11:string[])
      n7 = Index Array(array=w13, index=0) -> (element=→"Dependent Variable NAME" →"Dependent Variable NAME 2":string)
      n8 = Fract/Exp String To Number(string=w11) -> (number=→"ONLY Coefficients Array - Numeric":dbl[])  [unwired: 3 in, 1 out]
      n9 = Fract/Exp String To Number(string=w11) -> (number=w17:dbl[])  [unwired: 3 in, 1 out]
    }
    frame #1 {
      # "y = a0*y0 + a1*y1 + .....+ai*yi  \nwhere i =0 to 19.\ny0=1;\ny1=x1;\ny2=x2;              1st Order\ny3=x3;\n--------------\ny4=x1*x2;\ny5=x1*x3;\ny6=x2*x3;\ny7=x1**2;        2nd Order\ny8=x2**2;\ny9=x3**2;\n----------------\ny10=x1*x2*x3;\ny11=x1*x2**2;\ny12=x1*x3**2;\ny13=x2*x3**2;\ny14=x1**2*x2;  3rd Order\ny15=x1**2*x3;\ny16=x2**2*x3;\ny17=x1**3;\ny18=x2**3;\ny19=x3**3;"
      n10 = case shown="1" w23 {
        tunnel: w25 -> [_ w28 w45 w74]
        tunnel: [9999.0 ("y") w36 w59 w95] -> w26
        tunnel: w24 -> [_ w31 w58 w96]
        frame 0, Default {
        }
        frame 1 {
          n11 = Index Array(array=w28, index #1=0, index #2=1, index #3=2, index #4=3) -> (element #1=w40:dbl, element #2=w39:dbl, element #3=w38:dbl, element #4=w37:dbl)
          n12 = Index Array(array=w31, index #1=0, index #2=1, index #3=2) -> (element #1=w32:dbl, element #2=w30:dbl, element #3=w29:dbl)
          n13 = formula code="y=a0+a1*x1+a2*x2+a3*x3;"("a0"=w40, "a1"=w39, "a2"=w38, "a3"=w37, "x1"=w32, "x2"=w30, "x3"=w29) -> ("y"=w36:dbl)  [unwired: 3 out]
        }
        frame 2 {
          n14 = Index Array(array=w45, index #1=0, index #2=1, index #3=2, index #4=3, index #5=4, index #6=5, index #7=6, index #8=7, index #9=8, index #10=9) -> (element #1=w69:dbl, element #2=w68:dbl, element #3=w67:dbl, element #4=w66:dbl, element #5=w51:dbl, element #6=w50:dbl, element #7=w49:dbl, element #8=w48:dbl, element #9=w47:dbl, element #10=w46:dbl)
          n15 = Index Array(array=w58, index #1=0, index #2=1, index #3=2) -> (element #1=w62:dbl, element #2=w61:dbl, element #3=w60:dbl)
          n16 = formula code="y1=a0+a1*x1+a2*x2+a3*x3;\ny=y1+a4*x1*x2 + a5*x1*x3+a6*x2*x3+a7*x1**2+a8*x2**2+a9*x3**2;"("a0"=w69, "a1"=w68, "a2"=w67, "a3"=w66, "x1"=w62, "x2"=w61, "x3"=w60, "a4"=w51, "a5"=w50, "a6"=w49, "a7"=w48, "a8"=w47, "a9"=w46) -> ("y"=w59:dbl)  [unwired: 2 out]
        }
        frame 3 {
          n17 = Index Array(array=w74, index #1=0, index #2=1, index #3=2, index #4=3, index #5=4, index #6=5, index #7=6, index #8=7, index #9=8, index #10=9, index #11=10, index #12=11, index #13=12, index #14=13, index #15=14, index #16=15, index #17=16, index #18=17, index #19=18, index #20=19) -> (element #1=w118:dbl, element #2=w117:dbl, element #3=w116:dbl, element #4=w115:dbl, element #5=w102:dbl, element #6=w101:dbl, element #7=w100:dbl, element #8=w99:dbl, element #9=w98:dbl, element #10=w97:dbl, element #11=w84:dbl, element #12=w83:dbl, element #13=w82:dbl, element #14=w81:dbl, element #15=w80:dbl, element #16=w79:dbl, element #17=w78:dbl, element #18=w77:dbl, element #19=w76:dbl, element #20=w75:dbl)
          n18 = Index Array(array=w96, index #1=0, index #2=1, index #3=2) -> (element #1=w111:dbl, element #2=w110:dbl, element #3=w109:dbl)
          n19 = formula code="y1=a0+a1*x1+a2*x2+a3*x3;\ny2=y1+a4*x1*x2 + a5*x1*x3+a6*x2*x3+a7*x1**2+a8*x2**2+a9*x3**2;\ny3=y2+a10*x1*x2*x3+a11*x1*x2**2+a12*x1*x3**2+a13*x2*x3**2;\ny4=y3+a14*x1**2*x2+a15*x1**2*x3+a16*x2**2*x3+a17*x1**3;\ny=y4+a18*x2**3+a19*x3**3;"("a0"=w118, "a1"=w117, "a2"=w116, "a3"=w115, "x1"=w111, "x2"=w110, "x3"=w109, "a4"=w102, "a5"=w101, "a6"=w100, "a7"=w99, "a8"=w98, "a9"=w97, "a10"=w84, "a11"=w83, "a12"=w82, "a13"=w81, "a14"=w80, "a15"=w79, "a16"=w78, "a17"=w77, "a18"=w76, "a19"=w75) -> ("y"=w95:dbl)  [unwired: 4 out]
        }
      }
      "Calculated or Predicted VALUE" <- w26
    }
  }
